vi "TSM Relay Apply Configuration.vi"(0 "TSM Context":T1, 2 "Settling Time (0s)":dbl, 5 "Relay Configuration":tag, 11 "error in (no error)":errorcluster) -> (15 "error out":errorcluster)   [LabVIEW 2020]
doc: "Performs the actions specified by the relay configuration."
uses:
  <vilib>/NI_TestStand_SemiconductorModule/NI_TestStand_Semiconductor_Module.lvlibp/PinMap/General/SemiconductorModuleContext.ctl
  <vilib>/NI_TestStand_SemiconductorModule/NI_TestStand_Semiconductor_Module.lvlibp/PinMap/Relay Driver/ApplyRelayConfiguration.vi
  <vilib>/NI_TestStand_SemiconductorModule/NI_TestStand_Semiconductor_Module.lvlibp
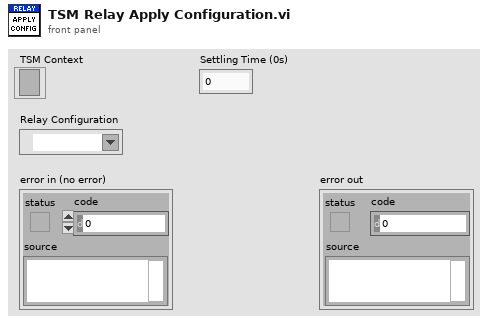
[diagram p1: front panel]
types:
  T1 = typedef "NI_TestStand_Semiconductor_Module.lvlibp/SemiconductorModuleContext.ctl" = refnum<k7>
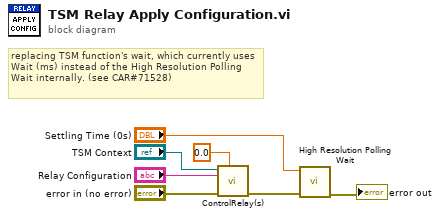
[diagram p0: block diagram]
diagram:
  # "replacing TSM function's wait, which currently uses Wait (ms) instead of the High Resolution Polling Wait internally. (see CAR#71528)"
  n1 = call-poly <vilib>:"ControlRelay(s).vi"("Wait (s)"=0.0, "error in (no error)"="error in (no error)", "Relay Configuration"="Relay Configuration", "Semiconductor Module Context"="TSM Context") -> ("error out"=w4:errorcluster)  [unwired: 6 in, 1 out]
  n2 = call <vilib>:"High Resolution Polling Wait.vi"("error in (no error)"=w4, "seconds to wait"="Settling Time (0s)") -> ("error out"=→"error out":errorcluster)  [unwired: 9 in]
